vi "moveMotorABS.vi"(8 "error in (no error)":errorcluster, 9 "Axis":enum16{"X", "Y"}(ring), 10 "L (mm)":dbl, 11 "VISA Refnum in":refnum<visa-resource-name>) -> (0 "error out":errorcluster, 3 "VISA Refnum out":refnum<visa-resource-name>)   [LabVIEW 2014]
doc: "Newport Motion Controler\nThis subVI move motor relative postion \n\nAndré Romero - 2020\nandretec@ifsc.usp.br"
uses:
  Global Motor Axis.vi
  <userlib>/Newport ESP301/Newport ESP301.lvlib
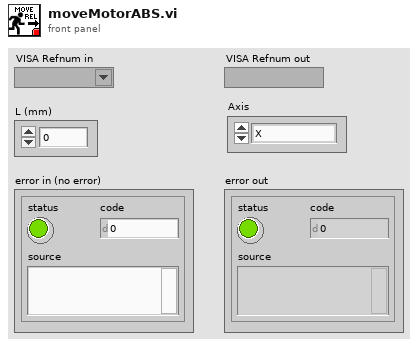
[diagram p1: front panel]
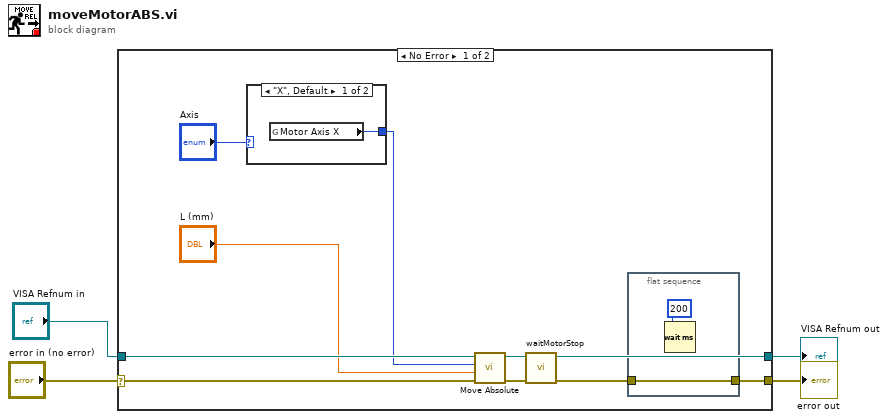
[diagram p0: block diagram]
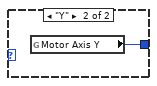
[diagram p2: hidden frame]
diagram:
  n1 = case shown="No Error" "error in (no error)" {
    selector: "error in (no error)" -> [w7 w19]
    tunnel: "VISA Refnum in" -> [w10 w20]
    tunnel: [w11 w19] -> w3
    tunnel: [w13 w20] -> w2
    frame No Error {
      n2 = case shown="\"X\", Default" "Axis" {
        tunnel: [w17 w18] -> w9
        frame "X", Default {
          n3 = global read "Global Motor Axis.vi" "Motor Axis X"() -> (w17:i32)
        }
        frame "Y" {
          n4 = global read "Global Motor Axis.vi" "Motor Axis Y"() -> (w18:i32)
        }
      }
      n5 = call <userlib>:"Move Absolute.vi"("error in (no error)"=w7, "Position (0 units)"="L (mm)", "Axis (1)"=w9, "VISA resource name"=w10) -> ("error out"=w6:errorcluster, "VISA resource name out"=w5:refnum<visa-resource-name>)  [unwired: 2 in]
      n6 = call "waitMotorStop.vi"("error in (no error)"=w6, "VISA Refnum in"=w5) -> ("error out"=w12:errorcluster, "VISA Refnum out"=w13:refnum<visa-resource-name>)  [unwired: 8 in]
      n7 = flat-sequence {
        tunnel: w12 -> [w16]
        tunnel: [w16] -> w11
        frame #0 {
          n8 = Wait (ms)(milliseconds to wait=u32 200) -> ()  [unwired: 1 out]
        }
      }
    }
    frame Error {
    }
  }
  "error out" <- w3
  "VISA Refnum out" <- w2
